vi "close_photosensor.vi"(8 "error in":errorcluster, 11 "task/channels in":refnum<k21>) -> (0 "error out":errorcluster)   [LabVIEW 2018]
doc: "This example demonstrates how to continuously acquire buffered voltage measurements using a DAQmx device.\n\nFor instructions on how to connect your signals to the DAQ device, refer to your device documentation."
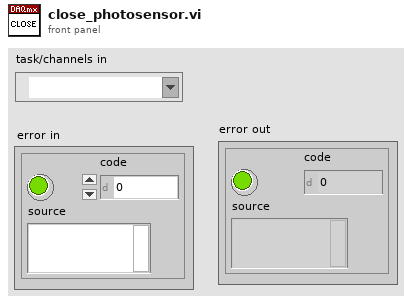
[diagram p1: front panel]
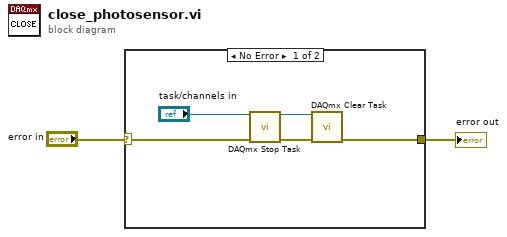
[diagram p0: block diagram]
diagram:
  n1 = case shown="No Error" "error in" {
    selector: "error in" -> [w4 w8]
    tunnel: [w3 w8] -> w1
    frame No Error {
      n2 = call "DAQmx Stop Task.vi"("task/channels in"="task/channels in", "error in"=w4) -> ("task out"=w6:refnum<k21>, "error out"=w7:errorcluster)  [unwired: 12 in]
      n3 = call "DAQmx Clear Task.vi"("task in"=w6, "error in"=w7) -> ("error out"=w3:errorcluster)  [unwired: 13 in]
    }
    frame Error {
    }
  }
  "error out" <- w1
